vi "WFRamp.vi"(8 "error in (no error)":errorcluster, 10 "Ramp Length (s)":dbl, 11 "Waveform In":waveform(dbl)) -> (0 "error out":errorcluster, 3 "Waveform Out":waveform(dbl))   [LabVIEW 2009]
uses:
  <vilib>/Waveform/WDTOps.llb/WDT Waveform Duration DBL.vi
  <vilib>/measure/NI_MABase.lvlib
  <vilib>/Waveform/WDTOps.llb/WDT Number of Waveform Samples DBL.vi
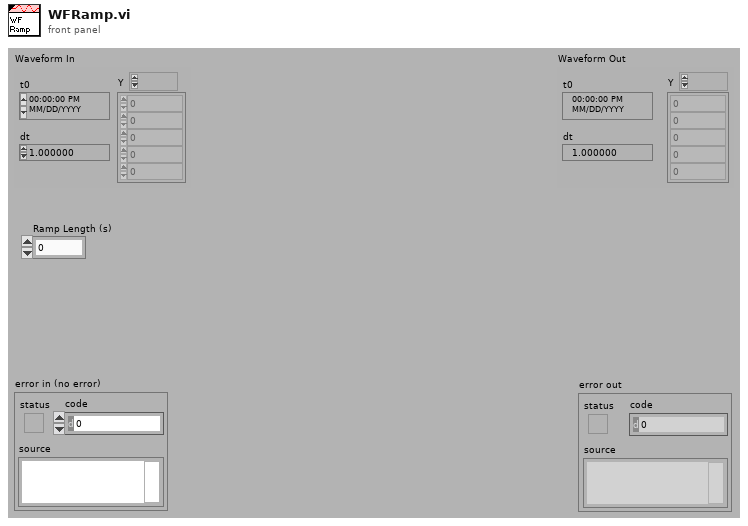
[diagram p1: front panel]
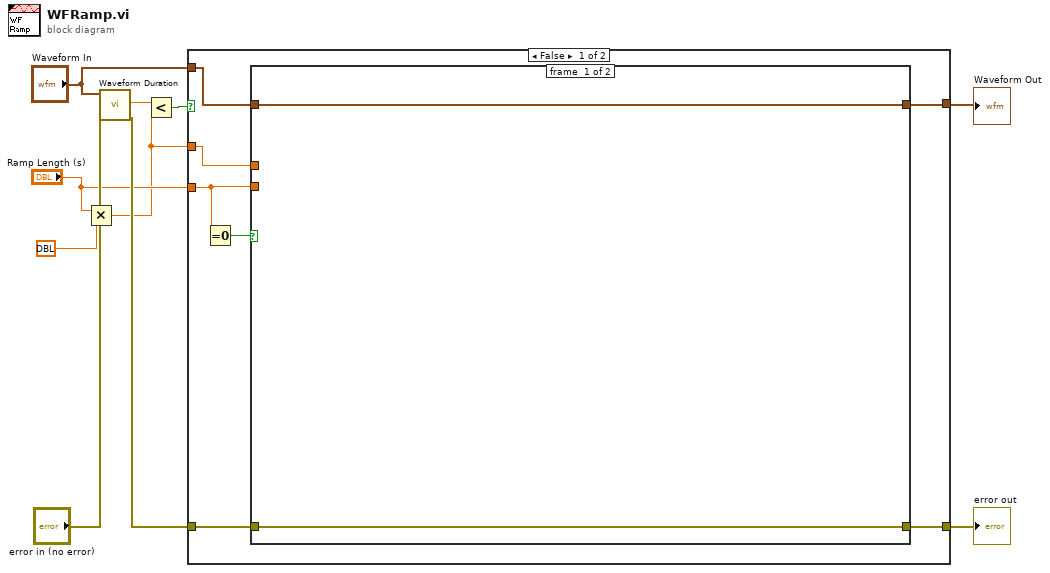
[diagram p0: block diagram]
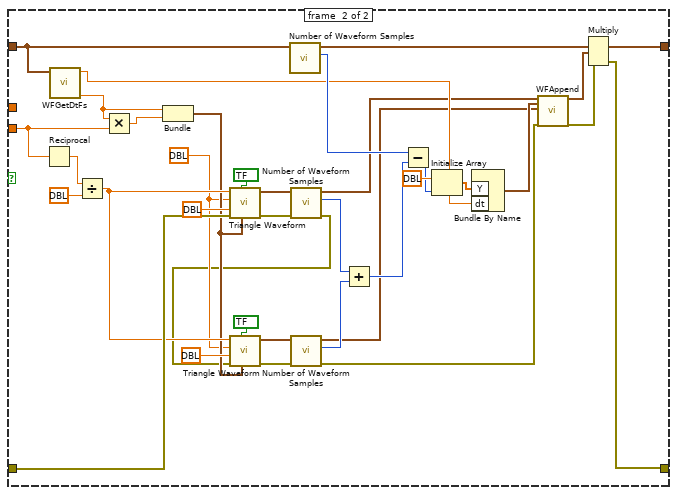
[diagram p2: hidden frame]
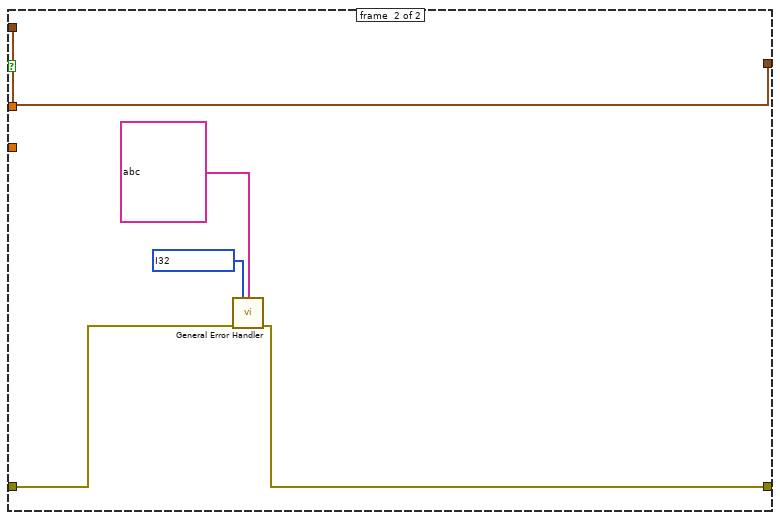
[diagram p3: hidden frame]
diagram:
  n1 = Multiply(x="Ramp Length (s)", y=dbl ?) -> (x*y=w2:dbl)
  n2 = call-poly <vilib>:"Waveform Duration.vi"("error in (no error)"="error in (no error)", "waveform in"="Waveform In") -> ("error out"=w8:errorcluster, "duration"=w1:dbl)  [unwired: 7 in, 1 out]
  n3 = Less?(x=w1, y=w2) -> (x < y?=w3:bool)
  n4 = case shown="False" w3 {
    tunnel: w8 -> [w17 w60]
    tunnel: [w13 w59] -> w5
    tunnel: "Waveform In" -> [w15 w56]
    tunnel: [w14 w56] -> w6
    tunnel: "Ramp Length (s)" -> [w11 _]
    tunnel: w2 -> [w16 _]
    frame #0 {
      n5 = Equal To 0?(x=w11) -> (x = 0?=w12:bool)
      n6 = case shown="False" w12 {
        tunnel: w17 -> [w18 w52]
        tunnel: w11 -> [_ w45]
        tunnel: w16 -> [_ _]
        tunnel: w15 -> [w19 w35]
        tunnel: [w19 w44] -> w14
        tunnel: [w18 w41] -> w13
        frame #0 {
        }
        frame #1 {
          w42 = dbl ? ("amplitude")
          n7 = Reciprocal(x=w45) -> (1/x=w55:dbl)
          n8 = call "WFGetDtFs.vi"("Waveform"=w35) -> ("Fs (Hz)"=w34:dbl, "dt"=w33:dbl)  [unwired: 9 in]
          n9 = Divide(x=w55, y=dbl ?) -> (x/y=w48:dbl)
          n10 = Multiply(x=w34, y=w45) -> (x*y=w51:dbl)
          n11 = Bundle("Fs (Hz)"=w34, w51) -> (w46:cluster{"Fs (Hz)":dbl, dbl})  [unwired: 1 in]
          n12 = call <vilib>:"Triangle Waveform.vi"("sampling info"=w46, "reset signal"=bool ?, "error in (no error)"=w52, "phase"=dbl ?, "amplitude"=w42, "frequency"=w48) -> ("error out"=w29:errorcluster, "signal out"=w31:waveform(dbl))  [unwired: 4 in]
          n13 = call-poly <vilib>:"Number of Waveform Samples.vi"("waveform in"=w35) -> ("number of samples"=w36:i32, "waveform out"=w37:waveform(dbl))  [unwired: 8 in, 1 out]
          n14 = call-poly <vilib>:"Number of Waveform Samples.vi"("error in (no error)"=w29, "waveform in"=w31) -> ("error out"=w28:errorcluster, "number of samples"=w26:i32, "waveform out"=w22:waveform(dbl))  [unwired: 7 in]
          n15 = call <vilib>:"Triangle Waveform.vi"("sampling info"=w46, "reset signal"=bool ?, "error in (no error)"=w28, "phase"=dbl ?, "amplitude"=w42, "frequency"=w48) -> ("error out"=w27:errorcluster, "signal out"=w30:waveform(dbl))  [unwired: 4 in]
          n16 = call-poly <vilib>:"Number of Waveform Samples.vi"("error in (no error)"=w27, "waveform in"=w30) -> ("error out"=w21:errorcluster, "number of samples"=w25:i32, "waveform out"=w23:waveform(dbl))  [unwired: 7 in]
          n17 = Add(x=w26, y=w25) -> (x+y=w24:i32)
          n18 = Subtract(x=w36, y=w24) -> (x-y=w20:i32)
          n19 = Initialize Array(dbl ? ("amplitude"), w20) -> (w43:dbl[])
          n20 = Bundle By Name("Y"=w43, "dt"=w33) -> (w38:waveform(dbl))  [unwired: 1 in]
          n21 = call "WFAppend.vi"("Waveform In"=w22, "Waveform In 2"=w38, "Waveform In 3"=w23, "error in (no error)"=w21) -> ("Waveform Out"=w40:waveform(dbl), "error out"=w39:errorcluster)  [unwired: 14 in]
          n22 = Multiply(1:w40, 2:w37, 4:w39) -> (0:w44:waveform(dbl), 3:w41:errorcluster)
        }
      }
    }
    frame #1 {
      n23 = call <vilib>:"General Error Handler.vi"("[user-defined codes]"=i32[] ?, "[user-defined descriptions]"=string[] ?, "error in (no error)"=w60) -> ("error out"=w59:errorcluster)  [unwired: 8 in, 4 out]
    }
  }
  "Waveform Out" <- w6
  "error out" <- w5
